vi "LVClass_ClosedLoopSecurityActivation_GetData.vi"(0 "ClosedLoopSecurity in":refnum<class "ClosedLoopSecurityActivation.lvclass">, 11 "error in (no error)":errorcluster) -> (4 "ClosedLoopSecurity out":refnum<class "ClosedLoopSecurityActivation.lvclass">, 6 "ClosedLoopSecurityActivationParams":T1, 15 "error out":errorcluster)   [LabVIEW 2020, in "ClosedLoopSecurityActivation.lvclass"]
doc: "get switches states\n\n<B>security_activationIn</B> : Pointer to Closed Loop activation params object.\n<B>security_activationOut</B> : Pointer to Closed Loop activation params object.\n<B>do_check_saturated_act_count</B> : Activates the requested actuators positions check, test will return false if\n too many acturators reach their boundaries\n<B>do_check_camera_fill_pct</B> : Activates the camera saturation level check\n<B>do_check_pupil_size_variation</B> : Activates the pupil size variation check, test will return false if pupil is\n too different from the interaction matrix pupil\n<B>do_check_dwf_pv</B> : Activates the delta wavefront peak-to-valley check"
uses:
  ClosedLoopSecurityActivation.lvclass
  ClosedLoopSecurityActivationParameters.ctl
  ClosedLoopSecurityActivation.lvclass/ClosedLoopSecurityActivation.ctl
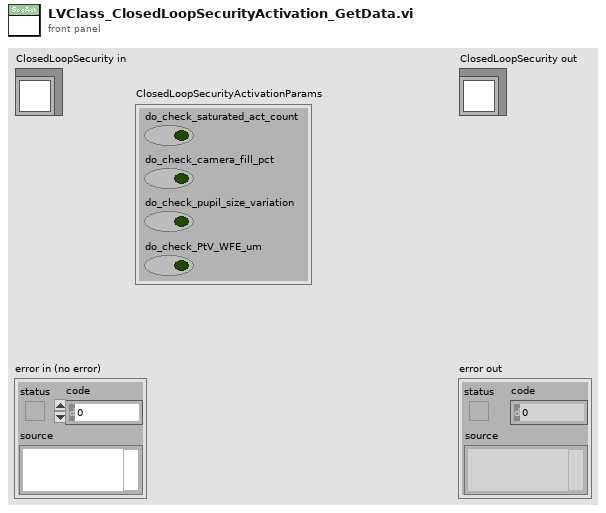
[diagram p1: front panel]
types:
  T1 = typedef "ClosedLoopSecurityActivationParameters.ctl" = cluster{"do_check_saturated_act_count":bool, "do_check_camera_fill_pct":bool, "do_check_pupil_size_variation":bool, "do_check_PtV_WFE_um":bool}
  T2 = typedef "ClassID.ctl" = i64
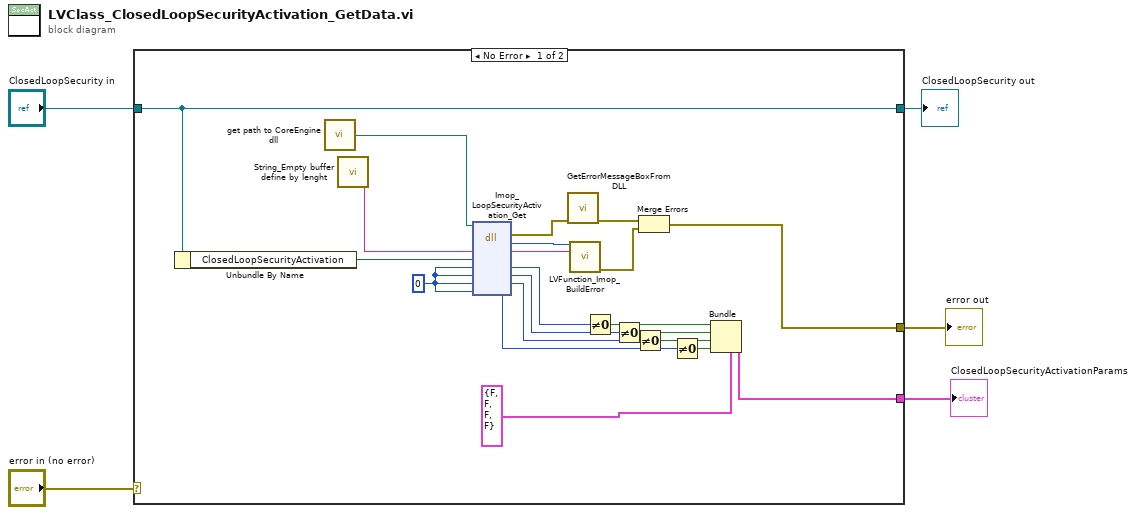
[diagram p0: block diagram]
diagram:
  n1 = case shown="No Error" "error in (no error)" {
    selector: "error in (no error)" -> [_ w28]
    tunnel: [w19 w28] -> w4
    tunnel: [w17 w27] -> w2
    tunnel: "ClosedLoopSecurity in" -> [w17 w27]
    tunnel: [w12 _] -> w1
    frame No Error {
      w6 = u8 0 ("High_amplitude")
      n2 = Unbundle By Name(w17) -> ("ClosedLoopSecurityActivation"=w18:T2)
      n3 = call "get path to CoreEngine dll.vi"() -> ("path to wavekit library"=w20:path)  [unwired: 14 in, 1 out]
      n4 = call "String_Empty buffer define by lenght.vi"() -> ("Empty buffer"=w26:string)  [unwired: 1 in]
      n5 = dll-call lib="D:/soft/HASO_v3/SVN_trunk/ImOpCoreEngine4_LV2011/DLLs/c_interface_vc100.dll" fn="Imop_LoopSecurityActivation_Get"(path in=w20, "message"=w26, "security_activation"=w18, "do_check_saturated_act_count"=w6, "do_check_camera_fill_pct"=w6, "do_check_pupil_size_variation"=w6, "do_check_loop_gain"=w6) -> (error out=w23:errorcluster, "return type"=w24:i32, "message"=w25:string, "do_check_saturated_act_count"=w16:u8, "do_check_camera_fill_pct"=w15:u8, "do_check_pupil_size_variation"=w14:u8, "do_check_loop_gain"=w13:u8)  [unwired: 3 in, 1 out]
      n6 = call "GetErrorMessageBoxFromDLL.vi"("error IN"=w23) -> ("error OUT"=w22:errorcluster)  [unwired: 10 in]
      n7 = call "LVFunction_Imop_BuildError.vi"("code"=w24, "String to Prepend to source (\"\")"=w25) -> ("error out"=w21:errorcluster)  [unwired: 13 in]
      n8 = Not Equal To 0?(x=w16) -> (x != 0?=w10:bool)
      n9 = Not Equal To 0?(x=w15) -> (x != 0?=w9:bool)
      n10 = Not Equal To 0?(x=w14) -> (x != 0?=w8:bool)
      n11 = Merge Errors(w22, w21) -> (w19:errorcluster)
      n12 = Not Equal To 0?(x=w13) -> (x != 0?=w7:bool)
      n13 = Bundle(cluster=T1 {"do_check_saturated_act_count"=FALSE, "do_check_camera_fill_pct"=FALSE, "do_check_pupil_size_variation"=FALSE, "do_check_PtV_WFE_um"=FALSE} ("ClosedLoopSecurityParams"), "do_check_saturated_act_count"=w10, "do_check_camera_fill_pct"=w9, "do_check_pupil_size_variation"=w8, "do_check_PtV_WFE_um"=w7) -> (w12:T1)
    }
    frame Error {
    }
  }
  "error out" <- w4
  "ClosedLoopSecurity out" <- w2
  "ClosedLoopSecurityActivationParams" <- w1
